vi "UpdateDatabase.vi"(3 "DatabaseIn":T1={"ExperimentDate"=timestamp(3449152041.4891562 s since 1904-01-01), "ImplantDate"=timestamp(3448288048.4255533 s since 1904-01-01), "CerebusFolder"="", "Experimenter"="Sara Hanrahan", "NHPName"="Frak", "DeviceType"="USEA", "DeviceSerial"="123456", "DeviceHemisphere"="Right", "DeviceRegion"="Median Nerve", "TaskType"="FingerMove", "TaskComments"="", "RecordingComments"="", "GeneralObservations"=""}, 4 "RecordsSelection":string="\u0000", 5 "CallType":enum16{"Initialize", "Save", "Load"}(ring)=enum."Save", 6 "DatabaseUDL":path=path "E:/Data/Setup2Database.udl") -> (0 "DatabaseOut":T1={"ExperimentDate"=timestamp(3401556199.892892 s since 1904-01-01), "ImplantDate"=timestamp(3401890063 s since 1904-01-01), "CerebusFolder"="", "Experimenter"="Tyler Davis", "NHPName"="201102", "DeviceType"="uECOG", "DeviceSerial"="CG-64BPX-F419", "DeviceHemisphere"="Right", "DeviceRegion"="Hand", "TaskType"="ArmMovementTask.vi", "TaskComments"="", "RecordingComments"="", "GeneralObservations"=""}, 1 "CerebusFoldersDates":string[](array[string]), 2 "ExperimentDatesSorted":string[](array[string]))   [LabVIEW 2012]
uses:
  <vilib>/addons/database/Connection.llb/DB Tools Open Connec (Path).vi
  <vilib>/addons/database/_DB Variant To Data/Database Variant To Data.xnode
  <vilib>/addons/database/NI_Database_API.lvlib
panel:
  out "Fields":string[](array[string])=["ExperimentDate", "ImplantDate", "CerebusFolder", "NHPName", "Experimenter", "DeviceType", "DeviceSerial", "DeviceHemisphere", "DeviceRegion", "TaskType", "TaskComments", "RecordingComments", "GeneralObservations"]
  out "ExperimentDates":string[](array[string])=["20130418-120000", "20111015-144319", "20111015-144319", "20111015-144319"]
  # "Do not place ';' or '=' in the comment fields"
  # "Do not place ';' or '=' in the comment fields"
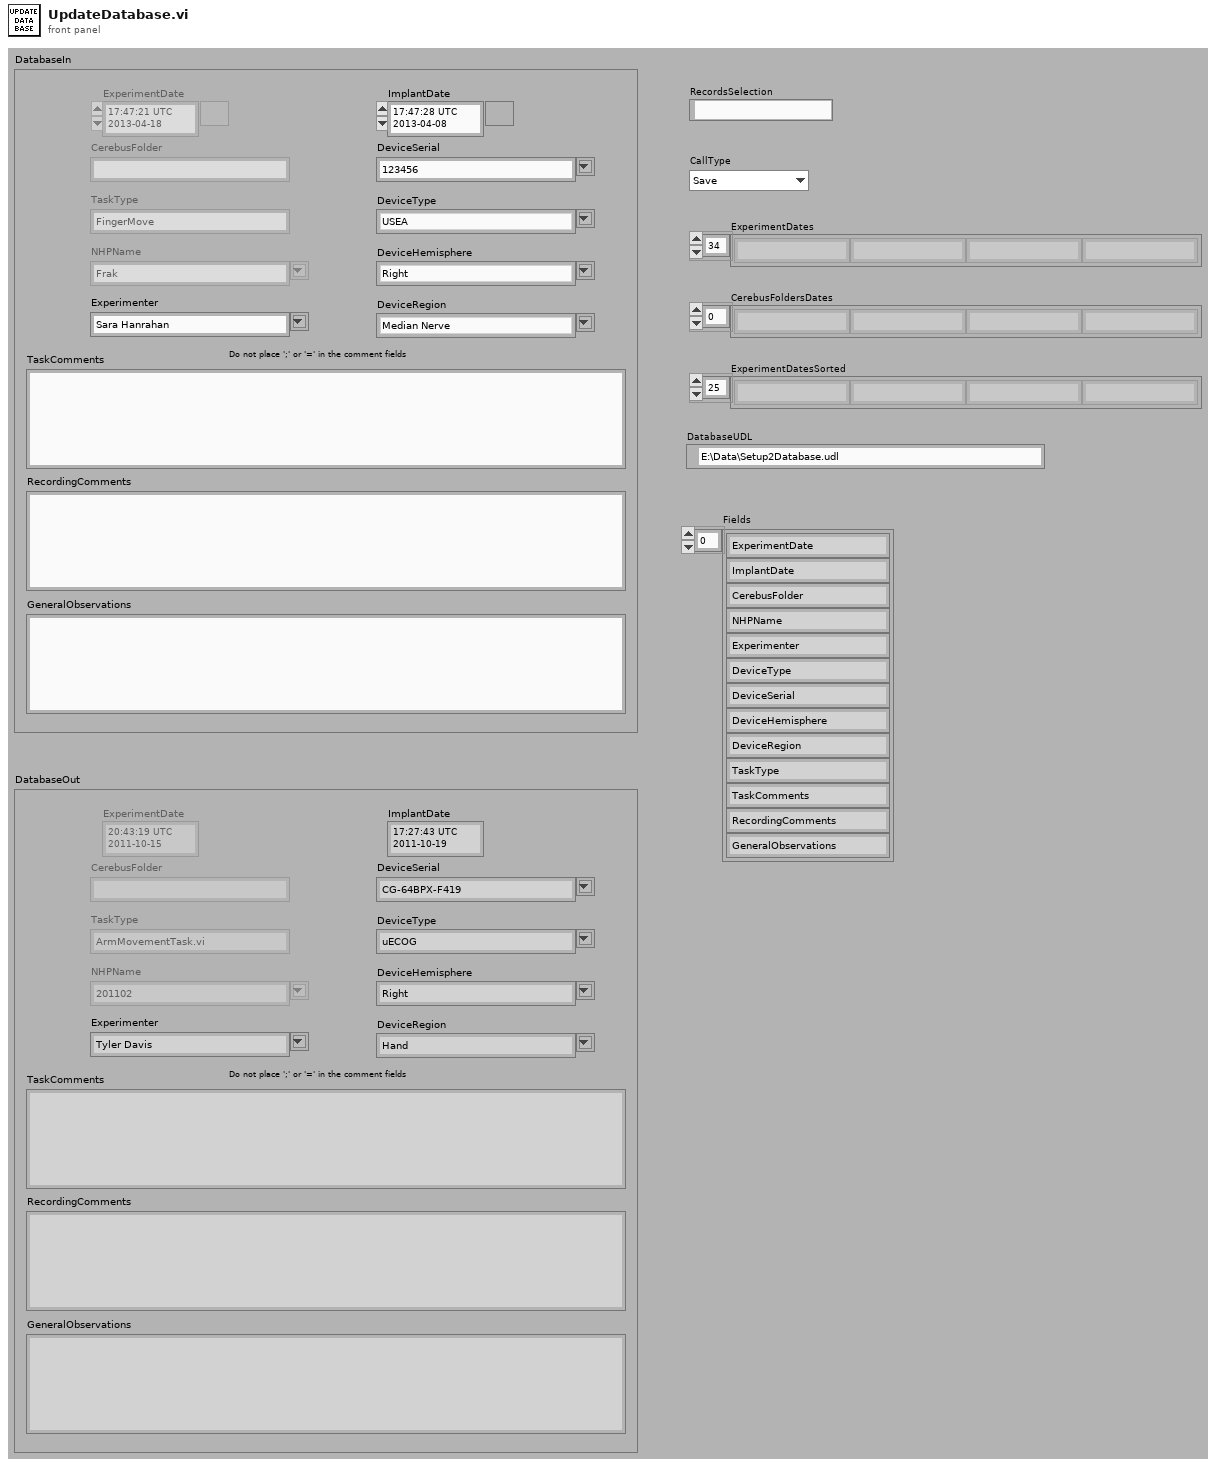
[diagram p1: front panel]
types:
  T1 = cluster{"ExperimentDate":timestamp, "ImplantDate":timestamp, "CerebusFolder":string, "Experimenter":string, "NHPName":string, "DeviceType":string, "DeviceSerial":string, "DeviceHemisphere":string, "DeviceRegion":string, "TaskType":string, "TaskComments":string, "RecordingComments":string, "GeneralObservations":string}
  T2 = typedef "NI_Database_API.lvlib/Conn ObjectReference.ctl" = refnum<k1>
  T3 = cluster{"data":timestamp, "data":timestamp, "data":string, "data":string, "data":string, "data":string, "data":string, "data":string, "data":string, "data":string, "data":string, "data":string, "data":string}
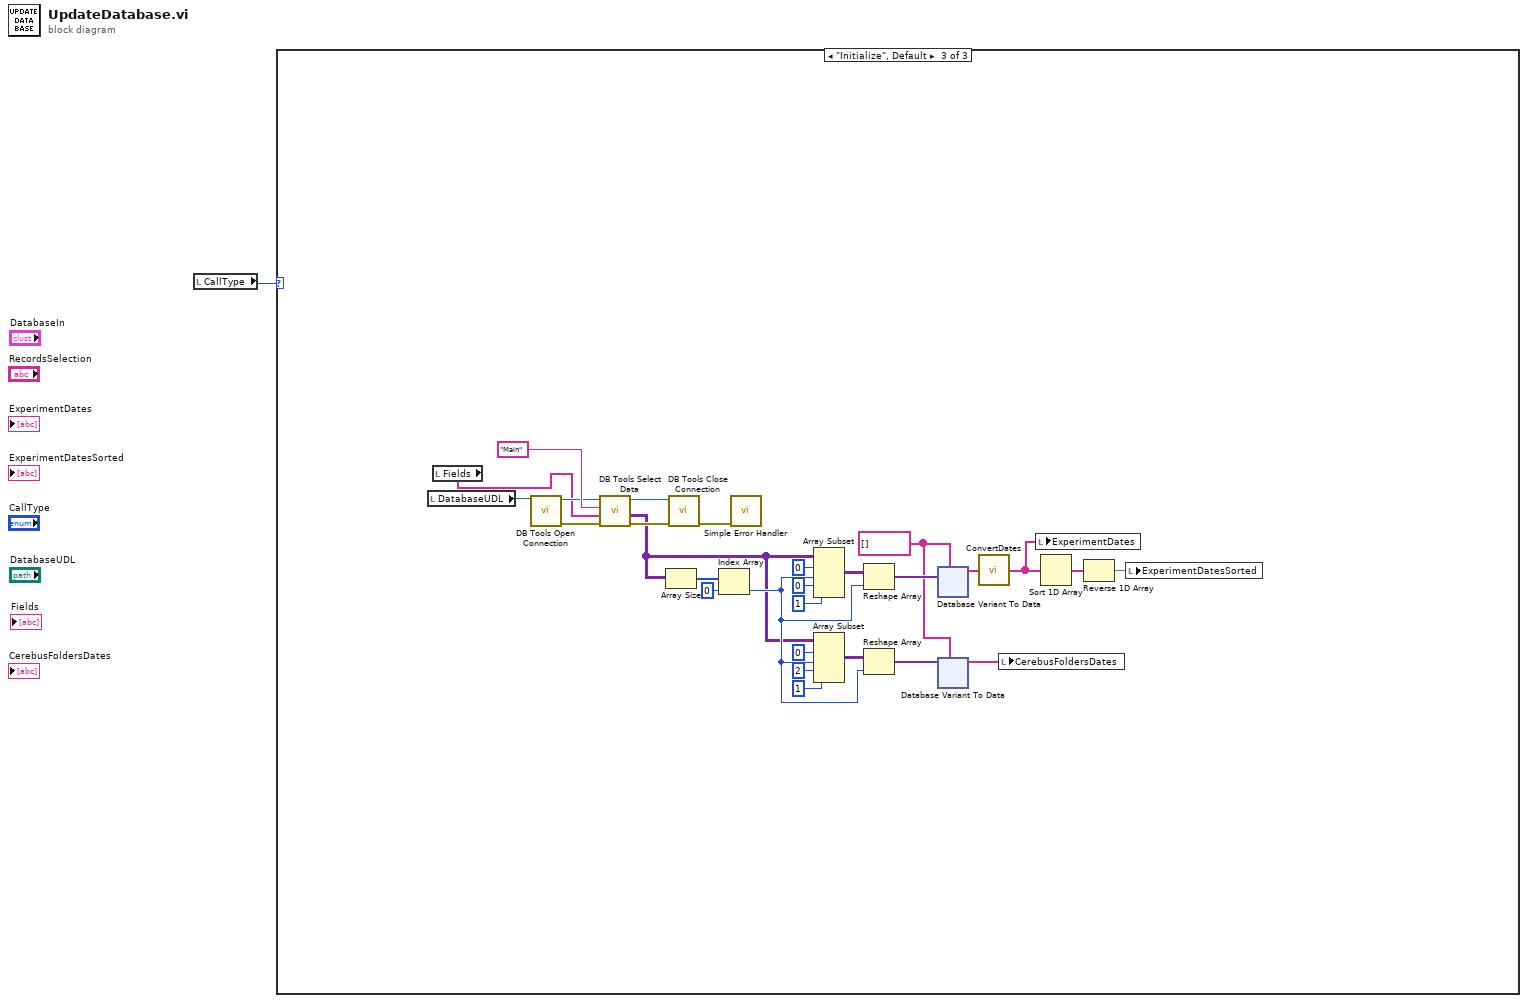
[diagram p0: block diagram]
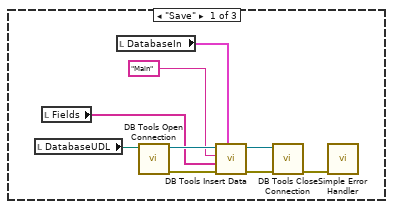
[diagram p2: hidden frame]
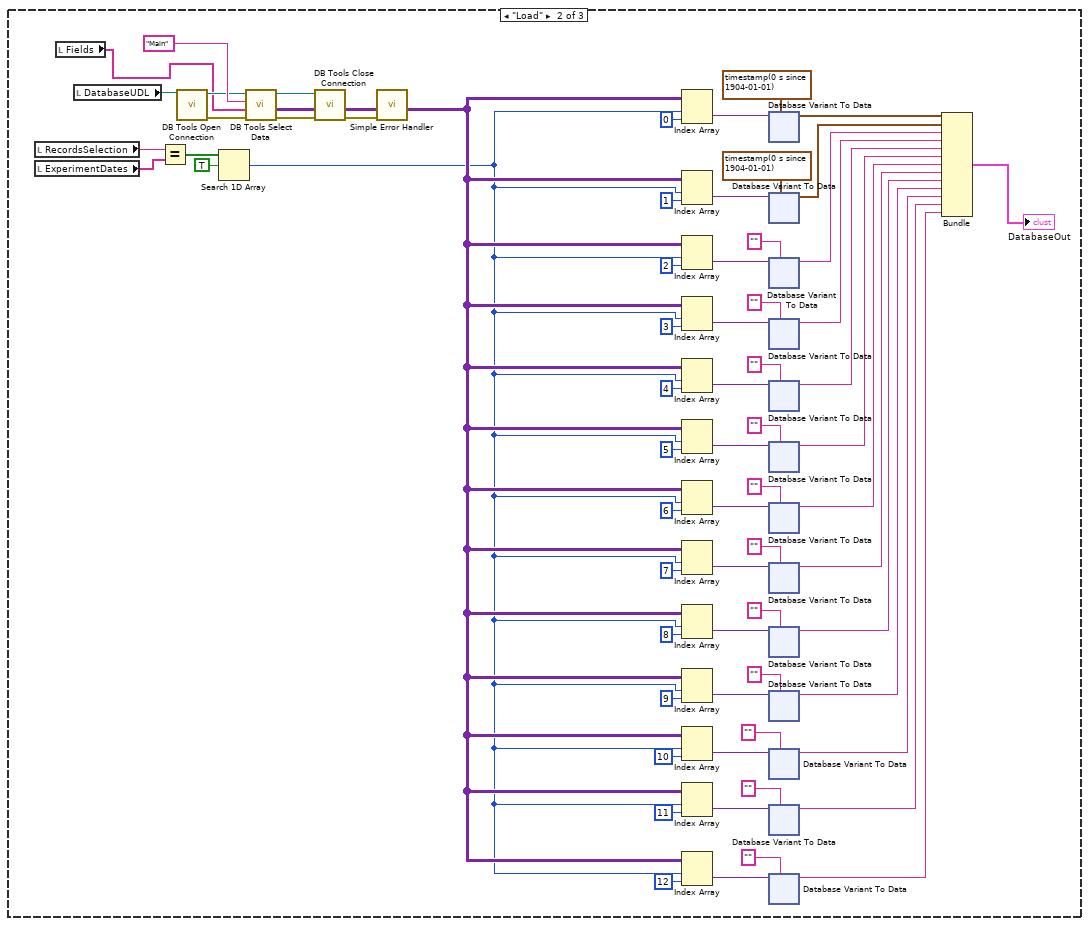
[diagram p3: hidden frame]
diagram:
  n1 = local read "CallType"() -> (w1:enum16{"Initialize", "Save", "Load"})
  n2 = case shown="\"Initialize\", Default" w1 {
    frame "Save" {
      n3 = local read "DatabaseUDL"() -> (w3:path)
      n4 = local read "Fields"() -> (w2:string[])
      n5 = local read "DatabaseIn"() -> (w4:T1)
      n6 = call-poly <vilib>:"DB Tools Open Connection.vi"("connection information"=w3) -> ("error out"=w8:errorcluster, "connection reference"=w10:T2)  [unwired: 7 in]
      n7 = call <vilib>:"DB Tools Insert Data.vi"("data"=w4, "error in (no error)"=w8, "columns"=w2, "table"="Main", "connection reference"=w10) -> ("error out"=w7:errorcluster, "connection reference out"=w6:T2)  [unwired: 5 in]
      n8 = call <vilib>:"DB Tools Close Connection.vi"("error in (no error)"=w7, "connection reference"=w6) -> ("error out"=w5:errorcluster)  [unwired: 5 in]
      n9 = call <vilib>:"Simple Error Handler.vi"("error in (no error)"=w5) -> ()  [unwired: 4 in, 5 out]
    }
    frame "Load" {
      n10 = local read "RecordsSelection"() -> (w29:string)
      n11 = local read "ExperimentDates"() -> (w28:string[])
      n12 = local read "Fields"() -> (w11:string[])
      n13 = local read "DatabaseUDL"() -> (w75:path)
      n14 = Equal?(x=w29, y=w28) -> (x = y?=w30:bool[])
      n15 = call-poly <vilib>:"DB Tools Open Connection.vi"("connection information"=w75) -> ("error out"=w77:errorcluster, "connection reference"=w71:T2)  [unwired: 7 in]
      n16 = Search 1D Array(1D array=w30, element=TRUE) -> (index of element=w13:i32)  [unwired: 1 in]
      n17 = call <vilib>:"DB Tools Select Data.vi"("error in (no error)"=w77, "columns"=w11, "table"="Main", "connection reference"=w71) -> ("error out"=w73:errorcluster, "data"=w14:variant[][], "connection reference out"=w72:T2)  [unwired: 2 in]
      n18 = call <vilib>:"DB Tools Close Connection.vi"("error in (no error)"=w73, "connection reference"=w72) -> ("error out"=w76:errorcluster)  [unwired: 5 in]
      n19 = call <vilib>:"Simple Error Handler.vi"("error in (no error)"=w76) -> ()  [unwired: 4 in, 5 out]
      n20 = Index Array(array=w14, index (row)=w13, index (col)=0 ("disabled index (col)")) -> (element=w69:variant)
      n21 = Index Array(array=w14, index (row)=w13, index (col)=1 ("disabled index (col)")) -> (element=w22:variant)
      n22 = Index Array(array=w14, index (row)=w13, index (col)=2 ("disabled index (col)")) -> (element=w67:variant)
      n23 = Index Array(array=w14, index (row)=w13, index (col)=3 ("disabled index (col)")) -> (element=w32:variant)
      n24 = Index Array(array=w14, index (row)=w13, index (col)=4 ("disabled index (col)")) -> (element=w62:variant)
      n25 = Index Array(array=w14, index (row)=w13, index (col)=5 ("disabled index (col)")) -> (element=w57:variant)
      n26 = Index Array(array=w14, index (row)=w13, index (col)=6 ("disabled index (col)")) -> (element=w56:variant)
      n27 = Index Array(array=w14, index (row)=w13, index (col)=7 ("disabled index (col)")) -> (element=w51:variant)
      n28 = Index Array(array=w14, index (row)=w13, index (col)=8 ("disabled index (col)")) -> (element=w50:variant)
      n29 = Index Array(array=w14, index (row)=w13, index (col)=9 ("disabled index (col)")) -> (element=w45:variant)
      n30 = Index Array(array=w14, index (row)=w13, index (col)=10 ("disabled index (col)")) -> (element=w44:variant)
      n31 = Index Array(array=w14, index (row)=w13, index (col)=11 ("disabled index (col)")) -> (element=w24:variant)
      n32 = Index Array(array=w14, index (row)=w13, index (col)=12 ("disabled index (col)")) -> (element=w18:variant)
      n33 = xnode "Database Variant To Data"("database variant"=w69, "type"=timestamp(0 s since 1904-01-01)) -> ("data"=w23:timestamp)  [unwired: 1 in, 1 out]
      n34 = xnode "Database Variant To Data"("database variant"=w22, "type"=timestamp(0 s since 1904-01-01)) -> ("data"=w20:timestamp)  [unwired: 1 in, 1 out]
      n35 = xnode "Database Variant To Data"("database variant"=w67, "type"="") -> ("data"=w42:string)  [unwired: 1 in, 1 out]
      n36 = xnode "Database Variant To Data"("database variant"=w32, "type"="") -> ("data"=w41:string)  [unwired: 1 in, 1 out]
      n37 = xnode "Database Variant To Data"("database variant"=w62, "type"="") -> ("data"=w40:string)  [unwired: 1 in, 1 out]
      n38 = xnode "Database Variant To Data"("database variant"=w57, "type"="") -> ("data"=w39:string)  [unwired: 1 in, 1 out]
      n39 = xnode "Database Variant To Data"("database variant"=w56, "type"="") -> ("data"=w38:string)  [unwired: 1 in, 1 out]
      n40 = xnode "Database Variant To Data"("database variant"=w51, "type"="") -> ("data"=w37:string)  [unwired: 1 in, 1 out]
      n41 = xnode "Database Variant To Data"("database variant"=w50, "type"="") -> ("data"=w36:string)  [unwired: 1 in, 1 out]
      n42 = xnode "Database Variant To Data"("database variant"=w45, "type"="") -> ("data"=w35:string)  [unwired: 1 in, 1 out]
      n43 = xnode "Database Variant To Data"("database variant"=w44, "type"="") -> ("data"=w34:string)  [unwired: 1 in, 1 out]
      n44 = xnode "Database Variant To Data"("database variant"=w24, "type"="") -> ("data"=w25:string)  [unwired: 1 in, 1 out]
      n45 = xnode "Database Variant To Data"("database variant"=w18, "type"="") -> ("data"=w15:string)  [unwired: 1 in, 1 out]
      n46 = Bundle("data"=w23, "data"=w20, "data"=w42, "data"=w41, "data"=w40, "data"=w39, "data"=w38, "data"=w37, "data"=w36, "data"=w35, "data"=w34, "data"=w25, "data"=w15) -> (→"DatabaseOut":T3)  [unwired: 1 in]
    }
    frame "Initialize", Default {
      w528 = string[] []
      n47 = local read "DatabaseUDL"() -> (w545:path)
      n48 = local read "Fields"() -> (w520:string[])
      n49 = call-poly <vilib>:"DB Tools Open Connection.vi"("connection information"=w545) -> ("error out"=w547:errorcluster, "connection reference"=w541:T2)  [unwired: 7 in]
      n50 = call <vilib>:"DB Tools Select Data.vi"("error in (no error)"=w547, "columns"=w520, "table"="Main", "connection reference"=w541) -> ("error out"=w543:errorcluster, "data"=w526:variant[][], "connection reference out"=w542:T2)  [unwired: 2 in]
      n51 = Array Size(array=w526) -> (size(s)=w539:i32[])
      n52 = call <vilib>:"DB Tools Close Connection.vi"("error in (no error)"=w543, "connection reference"=w542) -> ("error out"=w546:errorcluster)  [unwired: 5 in]
      n53 = Index Array(array=w539, index=0) -> (element=w529:i32)
      n54 = call <vilib>:"Simple Error Handler.vi"("error in (no error)"=w546) -> ()  [unwired: 4 in, 5 out]
      n55 = Array Subset(array=w526, index (row)=0 ("index"), length (row)=w529, index (col)=0 ("index"), length (col)=1 ("length")) -> (w535:variant[][])
      n56 = Array Subset(array=w526, index (row)=0 ("index"), length (row)=w529, index (col)=2 ("index"), length (col)=1 ("length")) -> (w533:variant[][])
      n57 = Reshape Array(w535, w529) -> (w534:variant[])
      n58 = Reshape Array(w533, w529) -> (w527:variant[])
      n59 = xnode "Database Variant To Data"("database variant"=w534, "type"=w528) -> ("data"=w522:string[])  [unwired: 1 in, 1 out]
      n60 = xnode "Database Variant To Data"("database variant"=w527, "type"=w528) -> ("data"=w525:string[])  [unwired: 1 in, 1 out]
      n61 = call "ConvertDates.vi"("Dates"=w522) -> ("ConvertedDates"=w521:string[])
      n62 = local write "CerebusFoldersDates"(w525) -> ()
      n63 = local write "ExperimentDates"(w521) -> ()
      n64 = Sort 1D Array(array=w521) -> (sorted array=w524:string[])
      n65 = Reverse 1D Array(array=w524) -> (reversed array=w523:string[])
      n66 = local write "ExperimentDatesSorted"(w523) -> ()
    }
  }
